vi "Sort Test Images.vi"(11 "path":path=path "C:/Users/Behavior Room/Desktop/Recordings/Single Mouse") -> (3 "Array":path[](array[path]))   [LabVIEW 2011]
uses:
  <vilib>/regexp/Match Regular Expression.xnode
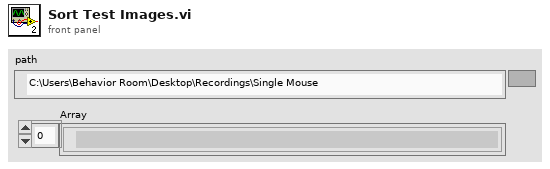
[diagram p1: front panel]
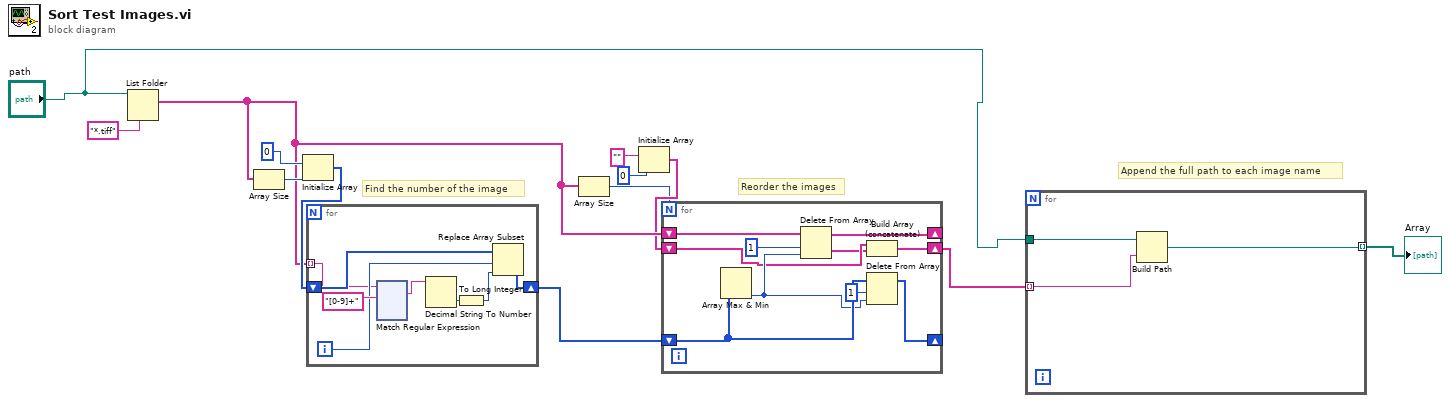
[diagram p0: block diagram]
diagram:
  # "Append the full path to each image name"
  # "Reorder the images"
  # "Find the number of the image"
  n1 = List Folder(path="path", pattern="*.tiff") -> (filenames=w7:string[])  [unwired: 2 in, 3 out]
  n2 = Array Size(array=w7) -> (size(s)=w12:i32)
  n3 = Initialize Array(0 ("index"), w12) -> (w10:i32[])
  n4 = for {
    tunnel: w7 -> [w14] mode=indexing
    shift-right: [w15] -> w9
    shift-left: w10 -> [w18]
    i -> [w17]
    n5 = xnode "Match Regular Expression"("input string"=w14, "regular expression"="[0-9]+") -> ("whole match"=w19:string)  [unwired: 4 in, 4 out]
    n6 = Decimal String To Number(string=w19) -> (number=w20:i32)  [unwired: 2 in, 1 out]
    n7 = To Long Integer(number=w20) -> (32bit integer=w16:i32)
    n8 = Replace Array Subset(array=w18, new element=w16, index=w17) -> (w15:i32[])
  }
  n9 = Array Size(array=w7) -> (size(s)=w5:i32)
  n10 = Initialize Array("" ("pattern"), 0 ("dimension size")) -> (w6:string[])
  n11 = for {
    N: w5 -> [_]
    shift-right: [w140] -> _
    shift-left: w9 -> [w142]
    shift-right: [w136] -> _
    shift-left: w7 -> [w137]
    shift-right: [w134] -> w3
    shift-left: w6 -> [w135]
    n12 = Array Max & Min(array=w142) -> (min index (indices)=w138:i32)  [unwired: 3 out]
    n13 = Delete From Array(array=w137, length=1, index=w138) -> (deleted portion=w133:string[], array with subset deleted=w136:string[])
    n14 = Build Array (concatenate)(w135, w133) -> (w134:string[])
    n15 = Delete From Array(array=w142, length=1, index=w138) -> (array with subset deleted=w140:i32[])  [unwired: 1 out]
  }
  n16 = for {
    tunnel: w3 -> [w144] mode=indexing
    tunnel: "path" -> [w145]
    tunnel: [w143] -> w1 mode=indexing
    n17 = Build Path(base path=w145, name or relative path=w144) -> (appended path=w143:path)
  }
  "Array" <- w1
